vi "synnax channel retrieve keys Array.vi"(0 "Synnax Client in":refnum<class "Synnax Client.lvclass">, 5 "channel names":string[](array[numeric]), 11 "error in":errorcluster) -> (4 "Synnax Client out":refnum<class "Synnax Client.lvclass">, 6 "channel keys":u32[](array[numeric]), 8 "data types":string[](array[numeric]), 10 "index keys":u32[](array[numeric]), 15 "error out":errorcluster)   [LabVIEW 2026, in "synnax_clib.lvlib" / "Synnax Client.lvclass"]
doc: "SYNNAX_EXPORT int32_t synnax_channel_retrieve_keys(\n SynnaxClient client,\n const char **names,\n uint64_t name_count,\n uint32_t *out_keys,\n SynnaxError err\n);"
uses:
  Synnax Client.lvclass
  Synnax Client.lvclass/Synnax Client.ctl
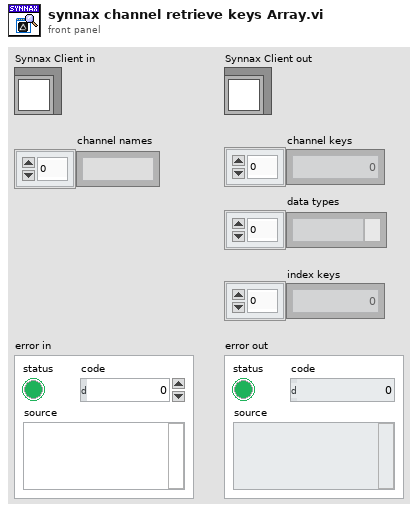
[diagram p1: front panel]
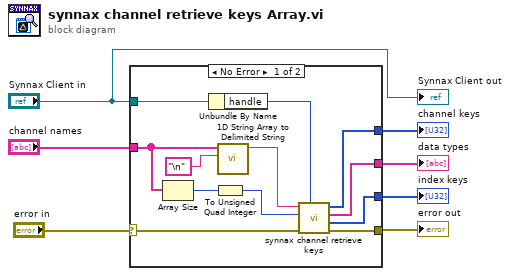
[diagram p0: block diagram]
diagram:
  n1 = case shown="No Error" "error in" {
    selector: "error in" -> [w9 w20]
    tunnel: "channel names" -> [w19 _]
    tunnel: "Synnax Client in" -> [w16 _]
    tunnel: [w15 _] -> w5
    tunnel: [w11 _] -> w4
    tunnel: [w10 w20] -> w3
    tunnel: [w8 _] -> w1
    frame No Error {
      n2 = Array Size(array=w19) -> (size(s)=w18:i32)
      n3 = Unbundle By Name(w16) -> ("handle"=w14:u64)
      n4 = To Unsigned Quad Integer(1:w18) -> (0:w12:u64)
      n5 = call <vilib>:"1D String Array to Delimited String.vi"("delimiter"="\n", "string array"=w19) -> ("delimited string"=w13:string)  [unwired: 9 in]
      n6 = call "synnax channel retrieve keys.vi"("handle"=w14, "error in (no error)"=w9, "count"=w12, "name(s)"=w13) -> ("error out"=w10:errorcluster, "out_index_keys"=w8:u32[], "out_dtypes"=w11:string[], "out_keys"=w15:u32[])  [unwired: 4 in]
    }
    frame Error {
    }
  }
  "channel keys" <- w5
  "data types" <- w4
  "error out" <- w3
  "index keys" <- w1
  "Synnax Client out" <- "Synnax Client in"
